vi "Search speed data file.vi"(8 "error in (no error)":errorcluster, 11 "Dummy AVI folder path":path) -> (0 "error out":errorcluster, 2 "Speed data file found":bool, 3 "1st speed data file's path":path)   [LabVIEW 2020]
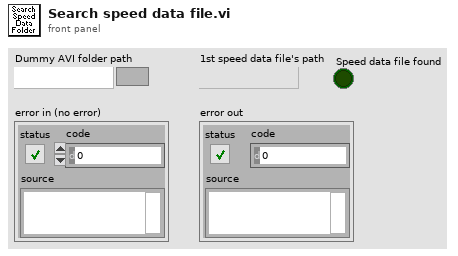
[diagram p1: front panel]
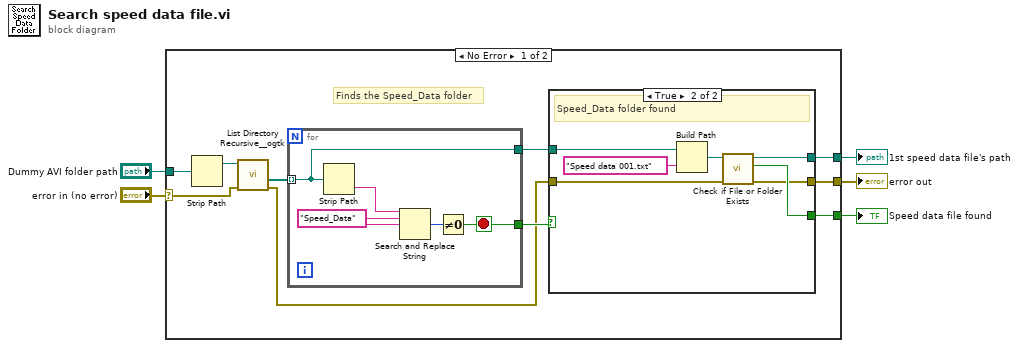
[diagram p0: block diagram]
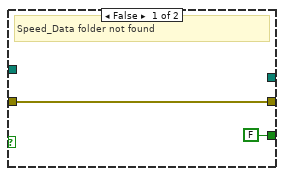
[diagram p2: hidden frame]
diagram:
  n1 = case shown="No Error" "error in (no error)" {
    selector: "error in (no error)" -> [w6 w30]
    tunnel: "Dummy AVI folder path" -> [w15 _]
    tunnel: [w11 _] -> w4
    tunnel: [w8 w30] -> w3
    tunnel: [w7 _] -> w2
    frame No Error {
      # "Finds the Speed_Data folder"
      n2 = Strip Path(path=w15) -> (stripped path=w14:path)  [unwired: 1 out]
      n3 = call <userlib>:"List Directory Recursive__ogtk.vi"("error in (no error)"=w6, "Path"=w14) -> ("error out"=w9:errorcluster, "dir paths"=w13:path[])  [unwired: 6 in, 2 out]
      n4 = for {
        tunnel: w13 -> [w26] mode=indexing
        tunnel: [w26] -> w10
        tunnel: [w25] -> w12
        stop <- w25 stop-if-true
        w28 = "Speed_Data" ("search string")
        n5 = Strip Path(path=w26) -> (name=w29:string)  [unwired: 1 out]
        n6 = Search and Replace String(input string=w29, search string=w28, replace string=w28) -> (number of replacements=w27:i32)  [unwired: 5 in, 3 out]
        n7 = Not Equal To 0?(x=w27) -> (x != 0?=w25:bool)
      }
      n8 = case shown="True" w12 {
        tunnel: [FALSE w21] -> w11
        tunnel: w10 -> [_ w24]
        tunnel: w9 -> [w16 w20]
        tunnel: [w16 w19] -> w8
        tunnel: [_ w18] -> w7
        frame False {
          # "Speed_Data folder not found"
        }
        frame True {
          # "Speed_Data folder found"
          n9 = Build Path(base path=w24, name or relative path="Speed data 001.txt" ("search string")) -> (appended path=w22:path)
          n10 = call <vilib>:"Check if File or Folder Exists.vi"("error in (no error)"=w20, "path"=w22) -> ("error out"=w19:errorcluster, "file or folder exists?"=w21:bool, "dup path"=w18:path)  [unwired: 7 in]
        }
      }
    }
    frame Error {
    }
  }
  "error out" <- w3
  "1st speed data file's path" <- w2
  "Speed data file found" <- w4
